vi "CounterCase.vi"() -> ()   [LabVIEW 2020]
doc: "8-bit counter with buttons for user. Version with while loop and cases. Comments in polish language."
panel:
  out "Num":bool[](array[boolean])
  out "TankOut":u8(slide) scale=0.0..255.0
  in  "Clear":bool
  out "NumOut":u8
  in  "Stop":bool
  in  "Dec":bool
  in  "Inc":bool
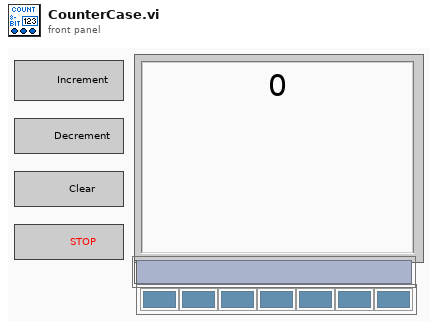
[diagram p1: front panel]
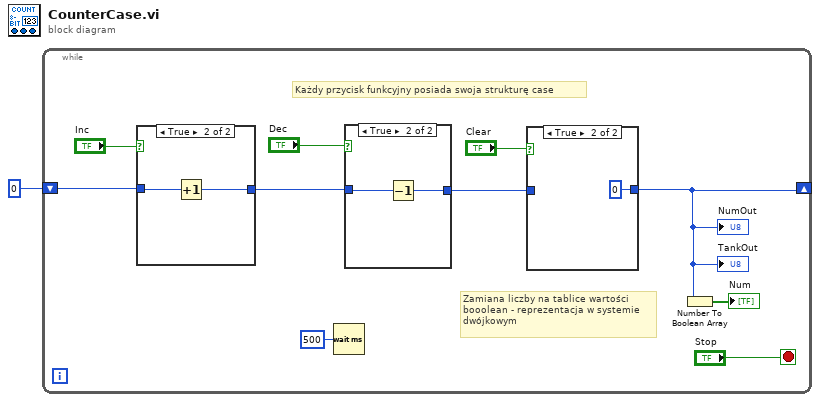
[diagram p0: block diagram]
diagram:
  n1 = while {
    shift-right: [w3] -> _
    shift-left: u8 0 -> [w9]
    stop <- "Stop" stop-if-true
    # "Zamiana liczby na tablice wartości\nbooolean - reprezentacja w systemie\ndwójkowym"
    # "Każdy przycisk funkcyjny posiada swoja strukturę case"
    n2 = case shown="True" "Inc" {
      tunnel: w9 -> [w17 w19]
      tunnel: [w17 w18] -> w7
      frame False {
      }
      frame True {
        n3 = Increment(x=w19) -> (x+1=w18:u8)
      }
    }
    n4 = Wait (ms)(milliseconds to wait=u32 500) -> ()  [unwired: 1 out]
    n5 = case shown="True" "Dec" {
      tunnel: w7 -> [w14 w16]
      tunnel: [w14 w15] -> w4
      frame False {
      }
      frame True {
        n6 = Decrement(x=w16) -> (x-1=w15:u8)
      }
    }
    n7 = case shown="True" "Clear" {
      tunnel: w4 -> [w12 _]
      tunnel: [w12 u8 0] -> w3
      frame False {
      }
      frame True {
      }
    }
    "NumOut" <- w3
    "TankOut" <- w3
    n8 = Number To Boolean Array(number=w3) -> (Boolean array=→"Num":bool[])
  }
